vi "GetParentTag.vi"(8 "ErrorIn(No Error)":errorcluster caption="entrée d'erreur (pas d'erreur)", 9 "LineNum":i32, 10 "Tag":string, 11 "TreeRef":refnum<vi>) -> (0 "sortie d'erreur":errorcluster, 1 "HasParent?":bool, 2 "Parent":string, 3 "TreeRefOut":refnum<vi>)   [LabVIEW 2019]
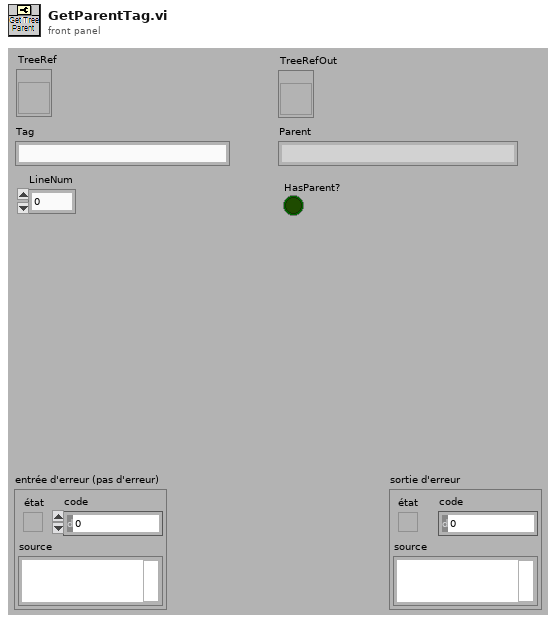
[diagram p1: front panel]
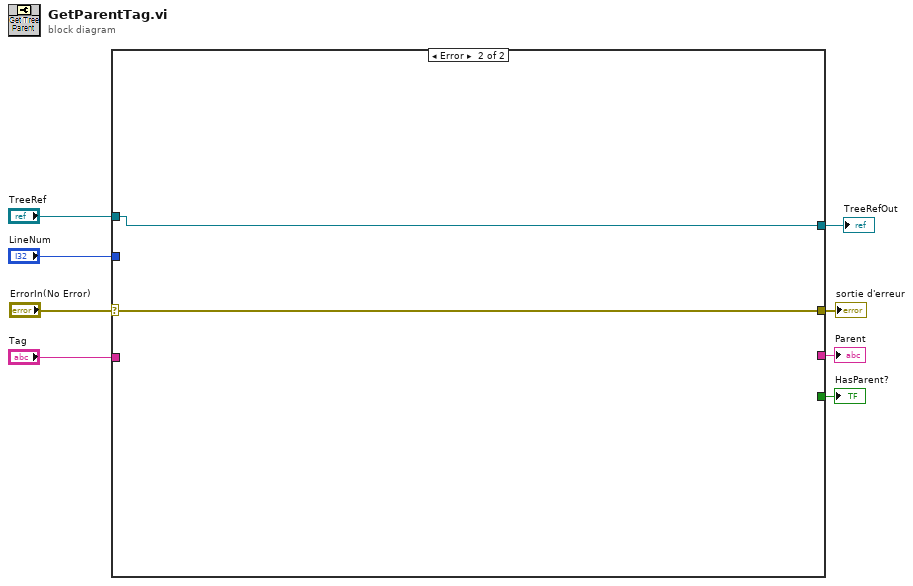
[diagram p0: block diagram]
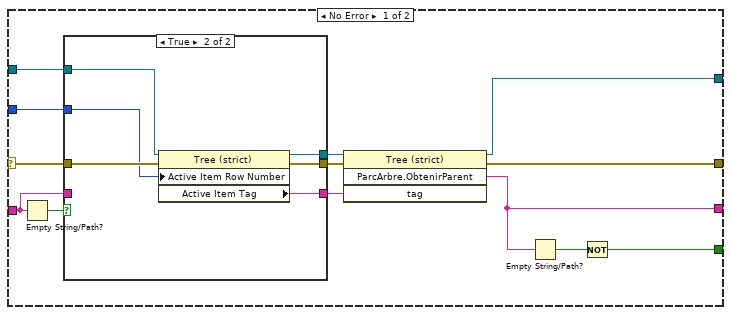
[diagram p2: hidden frame]
diagram:
  n1 = case shown="Error" "ErrorIn(No Error)" {
    selector: "ErrorIn(No Error)" -> [w19 w32]
    tunnel: [w18 w32] -> w7
    tunnel: "LineNum" -> [w17 _]
    tunnel: "TreeRef" -> [w16 w31]
    tunnel: [w12 _] -> w4
    tunnel: "Tag" -> [w13 _]
    tunnel: [w10 _] -> w2
    tunnel: [w9 w31] -> w1
    frame No Error {
      n2 = Empty String/Path?(string/path=w13) -> (empty?=w14:bool)
      n3 = case shown="True" w14 {
        tunnel: [w24 w30] -> w21
        tunnel: [w22 w29] -> w20
        tunnel: w19 -> [w22 w28]
        tunnel: w17 -> [_ w27]
        tunnel: w16 -> [w23 w26]
        tunnel: [w23 w25] -> w15
        tunnel: w13 -> [w24 _]
        frame False {
        }
        frame True {
          n4 = property on="Nœud de propriété" class="Tree (strict)"(reference=w26, error in=w28, "Active Item Row Number"=w27) -> (reference out=w25:refnum<vi>, error out=w29:errorcluster, "Active Item Tag"=w30:string)
        }
      }
      n5 = invoke on="Nœud de méthode" class="Tree (strict)" method="ParcArbre.ObtenirParent"(reference=w15, error in=w20, "tag"=w21) -> (reference out=w9:refnum<vi>, error out=w18:errorcluster, "Navigate Tree:Get Parent"=w12:string)  [unwired: 1 in, 1 out]
      n6 = Empty String/Path?(string/path=w12) -> (empty?=w11:bool)
      n7 = Not(x=w11) -> (.not. x?=w10:bool)
    }
    frame Error {
    }
  }
  "sortie d'erreur" <- w7
  "Parent" <- w4
  "HasParent?" <- w2
  "TreeRefOut" <- w1
